vi "Set_PS2_Volts.vi"(7 "delay (secs)":dbl=0.5 format="%#_13g", 8 "error in":errorcluster, 9 "Output on/off":bool=TRUE, 10 "Current Limit":dbl=0.75 min=0.0 max=6.0 format="%#.2g", 11 "Output Voltage":dbl format="%#_13g") -> (0 "error out":errorcluster, 2 "COM Port":string="COM16", 3 "Application Dir":path=path "C:/ModisEdge/Scanner/Test Sequence/ModisEdgeScanner.ini")   [LabVIEW 2015]
panel:
  in  "Maximum Output Voltage (31)":dbl=31.0 min=0.0 max=31.0 format="%#.2f"
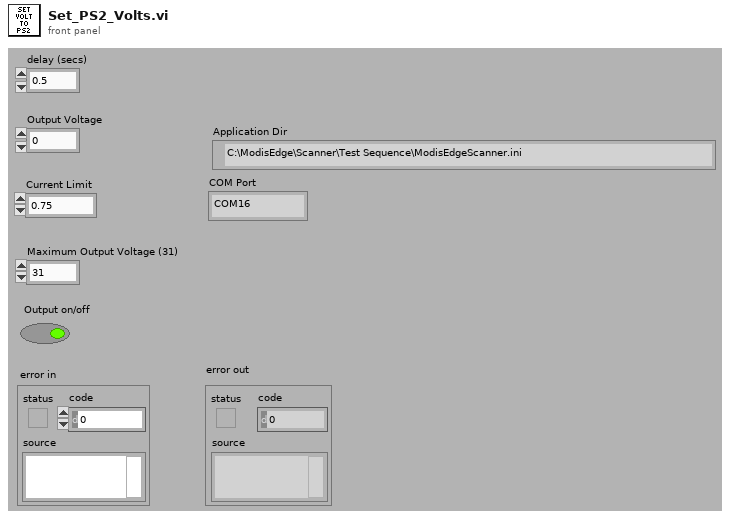
[diagram p1: front panel]
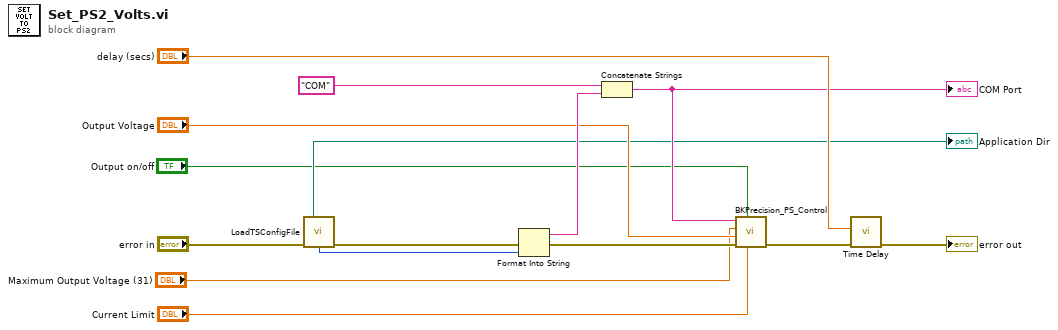
[diagram p0: block diagram]
diagram:
  n1 = call "LoadTSConfigFile.vi"("error in (no error)"="error in") -> ("appended path"=→"Application Dir":path, "PS2_COMPort"=w6:i32, "error out"=w4:errorcluster)  [unwired: 4 in, 8 out]
  n2 = Format Into String(error in=w4, w6) -> (resulting string=w14:string, error out=w9:errorcluster)  [unwired: 2 in]
  n3 = Concatenate Strings("COM" ("string"), w14) -> (w11:string)
  "COM Port" <- w11
  n4 = call "BKPrecision_PS_Control.vi"("Current Limit (0)"="Current Limit", "Output on/off"="Output on/off", "error in (no error)"=w9, "Output Voltage (0)"="Output Voltage", "Maximum Output Voltage (31)"="Maximum Output Voltage (31)", "VISA resource name"=w11) -> ("error out"=w8:errorcluster)  [unwired: 4 in, 1 out]
  n5 = call "Time Delay"("error in (no error)"=w8, "Delay Time (s)"="delay (secs)") -> ("error out"=→"error out":errorcluster)  [unwired: 9 in]
